vi "get_digital_output_values.vi"(0 "reference (in)":i32, 2 "do (single)":T1, 4 "get_all? (def=F)":bool, 5 "error in (no error)":errorcluster) -> (14 "reference (dup)":i32, 15 "dig_out_val (single only)":bool, 16 "do_items":T2[](array[typedef]), 17 "raw_do_value":string, 19 "error out":errorcluster)   [LabVIEW 2012]
doc: "This VI reads the state of all the device's digital outputs. The developer is given the choice to retrieve ALL the states or only the state of a single channel. To retrieve all, be sure the \"get_all?\" boolean is set to TRUE. To get just one, be sure to select the appropriate item the in \"do (single)\" input.\n\nProduced By:\n\nChristopher Lemieux\nKod Integrations, LLC\n4835 Marianne Drive\nMount Airy, MD 21771\nhttp://www.kodintegrations.com\nemail: clemieux@kodintegrations.com\nphone: (240) 687-1288"
uses:
  support/controls/digital_output_item_group.ctl
  support/controls/digital_output_items.ctl
  main_functions/commands.ctl
  support/controls/simple_actions.ctl
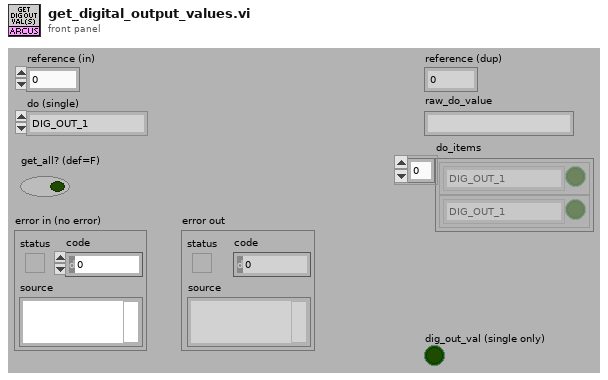
[diagram p1: front panel]
types:
  T1 = typedef "digital_output_items.ctl" = enum16{"DIG_OUT_1", "DIG_OUT_2"}
  T2 = typedef "digital_output_item_group.ctl" = cluster{"item":T1, "status":bool}
  T3 = typedef "commands.ctl" = enum16{"clear error", "constant jog(-)", "constant jog(+)", "get acceleration", "get actual current", "get device id", "get digital input status", "get digial inputs status", "get dig output status", "get digital outputs status", "get firmware ver", "get high speed", "get idle current", "get low speed", "get micro step", "get motor status", "get move mode", "get polarity", "get position", "get product id", "get power status", "get run current", "get status", "home(-)", "home(+)", "move to position", "power down", "power up", "set acceleration", "set device id", "set digital output", "set digital outputs", "set high speed", "set idle current", "set low speed", "set move mode absolute", "set move mode increment", "set polarity", "set position", "set run current", "stop immediate", "stop slow", "store to memory"}
  T4 = typedef "simple_actions.ctl" = enum16{"from", "to"}
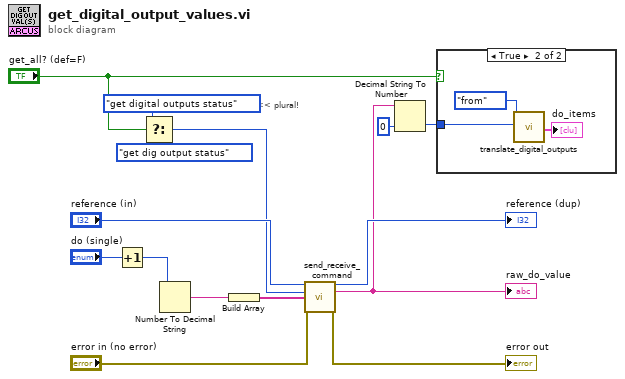
[diagram p0: block diagram]
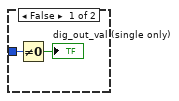
[diagram p2: hidden frame]
diagram:
  # "<<< plural!"
  n1 = Increment(x="do (single)") -> (x+1=w1:T1)
  n2 = Select(t=commands."get digital outputs status" ("command"), s="get_all? (def=F)", f=commands."get dig output status" ("command")) -> (s? t:f=w7:T3)
  n3 = Number To Decimal String(number=w1) -> (decimal integer string=w2:string)  [unwired: 1 in]
  n4 = Build Array(w2) -> (w3:string[])
  n5 = call "send_receive_command.vi"("reference (in)"="reference (in)", "command"=w7, "params (opt)"=w3, "error in (no error)"="error in (no error)") -> ("reference (dup)"=→"reference (dup)":i32, "read_string"=w13:string, "error out"=→"error out":errorcluster)  [unwired: 7 in, 2 out]
  "raw_do_value" <- w13
  n6 = Decimal String To Number(string=w13, default (0L)=u32 0 ("default (0 I32)")) -> (number=w6:u32)  [unwired: 1 in, 1 out]
  n7 = case shown="True" "get_all? (def=F)" {
    tunnel: w6 -> [w17 w20]
    frame False {
      n8 = Not Equal To 0?(x=w17) -> (x != 0?=→"dig_out_val (single only)":bool)
    }
    frame True {
      n9 = call "translate_digital_outputs.vi"("simple_actions"=simple_actions."from", "do_value (in)"=w20) -> ("digital_output_items (out)"=→"do_items":T2[])  [unwired: 16 in, 1 out]
    }
  }
